vi "LVOBJ Find.vi"(10 "Key":string, 11 "Values":T1[](array[typedef])) -> (2 "Found?":bool, 3 "Value":T1)   [LabVIEW 2019, in "labview_json.lvlib"]
uses:
  labview_json.lvlib
  Value.ctl
  Value Type.ctl
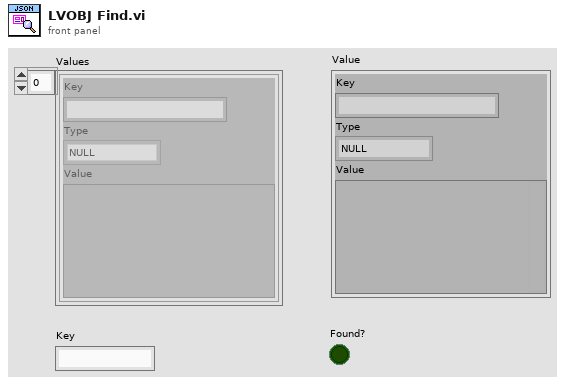
[diagram p1: front panel]
types:
  T1 = typedef "labview_json.lvlib/Value.ctl" = cluster{"Key":string, "Type":T2, "Value":variant}
  T2 = typedef "labview_json.lvlib/Value Type.ctl" = enum8{"NULL", "OBJECT", "ARRAY", "BOOL", "INT", "UINT", "FLOAT", "STRING"}
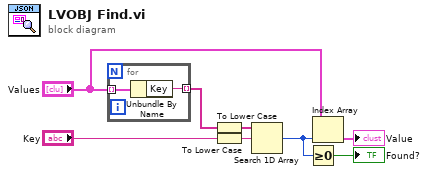
[diagram p0: block diagram]
diagram:
  n1 = for {
    tunnel: "Values" -> [w10] mode=indexing
    tunnel: [w9] -> w8 mode=indexing
    n2 = Unbundle By Name(w10) -> ("Key"=w9:string)
  }
  n3 = To Lower Case(string=w8) -> (all lower case string=w6:string[])
  n4 = To Lower Case(string="Key") -> (all lower case string=w5:string)
  n5 = Search 1D Array(1D array=w6, element=w5) -> (index of element=w3:i32)  [unwired: 1 in]
  n6 = Greater Or Equal To 0?(x=w3) -> (x >= 0?=→"Found?":bool)
  n7 = Index Array(array="Values", index=w3) -> (element=→"Value":T1)
